vi "rhominusdot_growth.vi"(5 "rho- sat in":dbl[](array[numeric]), 7 "rho+ sat in":dbl[](array[numeric]), 8 "Sat pol in":dbl, 9 "rho- in":dbl[](array[numeric]), 10 "rho0 in":dbl[](array[numeric]), 11 "rho+ in":dbl[](array[numeric])) -> (3 "rho- dot out":dbl[](array[numeric]))   [LabVIEW 2018]
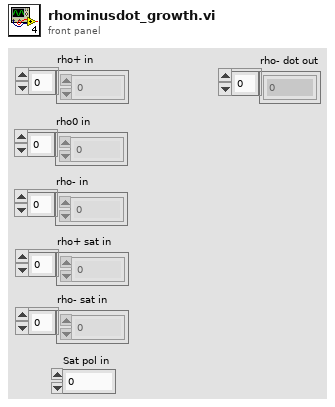
[diagram p1: front panel]
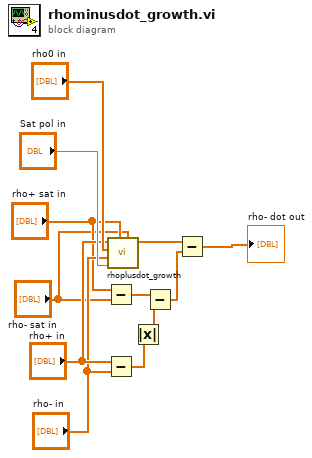
[diagram p0: block diagram]
diagram:
  n1 = Subtract(x="rho+ sat in", y="rho- sat in") -> (x-y=w12:dbl[])
  n2 = Subtract(x="rho+ in", y="rho- in") -> (x-y=w11:dbl[])
  n3 = call "rhoplusdot_growth.vi"("rho- sat in"="rho- sat in", "rho+ sat in"="rho+ sat in", "Sat pol in"="Sat pol in", "rho- in"="rho- in", "rho0 in"="rho0 in", "rho+ in"="rho+ in") -> ("rho+ dot out"=w4:dbl[])  [unwired: 5 in]
  n4 = Absolute Value(x=w11) -> (abs(x)=w1:dbl[])
  n5 = Subtract(x=w12, y=w1) -> (x-y=w2:dbl[])
  n6 = Subtract(x=w4, y=w2) -> (x-y=→"rho- dot out":dbl[])
